vi "elements table.vi"(6 "error in (no error)":errorcluster, 9 "A/D":enum16{"Analogico", "Digital"}(ring)) -> (0 "error out":errorcluster, 3 "x+y":i32)   [LabVIEW 2020, in "Settings.lvlib"]
uses:
  Settings.lvlib
  <vilib>/drjdpowell/SQLite Library/SQL Connection/Open (path).vi
  <vilib>/drjdpowell/SQLite Library/SQL Connection/Open (string).vi
  <vilib>/AdvancedString/Path To Command Line String.vi
  <vilib>/drjdpowell/SQLite Library/SQL Connection/Execute SQL.vi
  <vilib>/drjdpowell/SQLite Library/SQL Connection/Connection.lvclass
  <vilib>/drjdpowell/SQLite Library/SQLite.lvlib
panel:
  out "Numeric 2":i32
  out "Numeric":i32
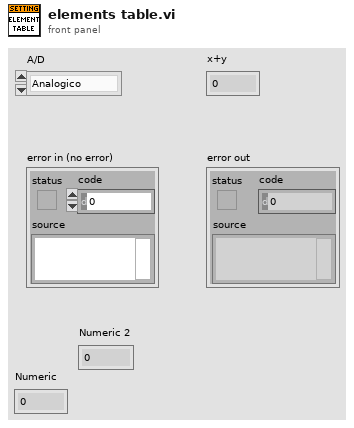
[diagram p1: front panel]
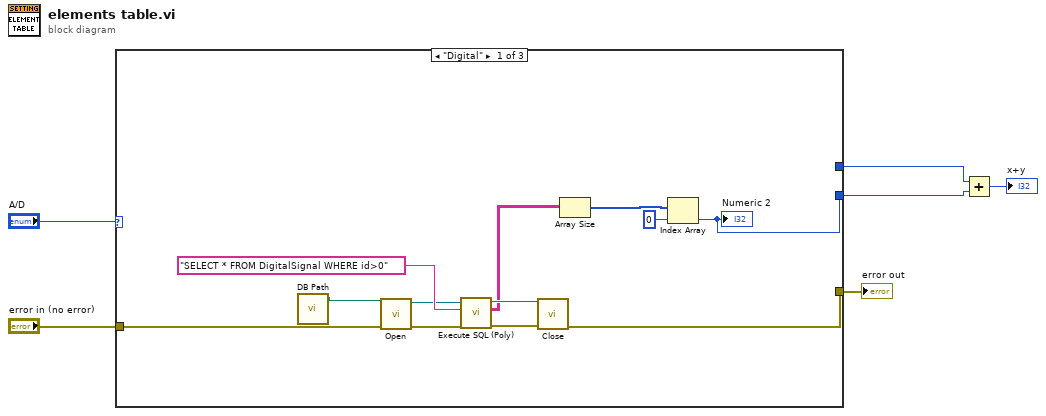
[diagram p0: block diagram]
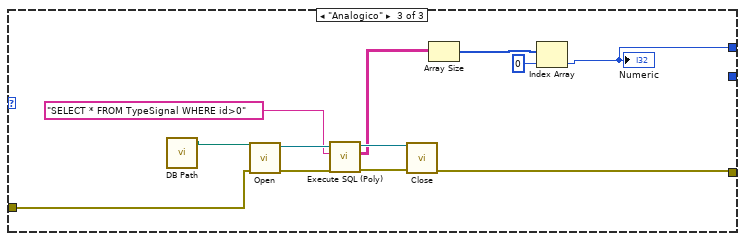
[diagram p3: hidden frame]
diagram:
  n1 = case shown="\"Digital\"" "A/D" {
    tunnel: [w11 w19 w25] -> w6
    tunnel: "error in (no error)" -> [w12 w19 w26]
    tunnel: [_ _ w20] -> w2
    tunnel: [w7 _ _] -> w1
    frame "Digital" {
      n2 = call "DB Path.vi"() -> ("DB path"=w18:path)  [unwired: 11 in]
      n3 = call-poly <vilib>:"Open.vi"("error in (no error)"=w12, "db file"=w18) -> ("error out"=w13:errorcluster, "SQLite Connection"=w14:refnum<class "Connection.lvclass">)  [unwired: 8 in]
      n4 = call-poly <vilib>:"Execute SQL (Poly).vi"("error in (no error)"=w13, "SQL"="SELECT * FROM DigitalSignal WHERE id>0", "SQLite Connection in"=w14) -> ("error out"=w16:errorcluster, "Result Set"=w10:string[][], "SQLite Connection"=w15:refnum<class "Connection.lvclass">)  [unwired: 5 in, 1 out]
      n5 = call-dynamic "Close.vi"("error in (no error)"=w16, "SQLite Connection in"=w15) -> ("error out"=w11:errorcluster)  [unwired: 9 in]
      n6 = Array Size(array=w10) -> (size(s)=w8:i32[])
      n7 = Index Array(array=w8, index=0) -> (element=w7:i32)
      "Numeric 2" <- w7
    }
    frame Default {
    }
    frame "Analogico" {
      n8 = call "DB Path.vi"() -> ("DB path"=w31:path)  [unwired: 11 in]
      n9 = call-poly <vilib>:"Open.vi"("error in (no error)"=w26, "db file"=w31) -> ("error out"=w27:errorcluster, "SQLite Connection"=w28:refnum<class "Connection.lvclass">)  [unwired: 8 in]
      n10 = call-poly <vilib>:"Execute SQL (Poly).vi"("error in (no error)"=w27, "SQL"="SELECT * FROM TypeSignal WHERE id>0", "SQLite Connection in"=w28) -> ("error out"=w30:errorcluster, "Result Set"=w24:string[][], "SQLite Connection"=w29:refnum<class "Connection.lvclass">)  [unwired: 5 in, 1 out]
      n11 = call-dynamic "Close.vi"("error in (no error)"=w30, "SQLite Connection in"=w29) -> ("error out"=w25:errorcluster)  [unwired: 9 in]
      n12 = Array Size(array=w24) -> (size(s)=w21:i32[])
      n13 = Index Array(array=w21, index=0) -> (element=w20:i32)
      "Numeric" <- w20
    }
  }
  "error out" <- w6
  n14 = Add(x=w2, y=w1) -> (x+y=→"x+y":i32)
